vi "__uintAdd.vi"(8 "Base (decimal)":T1=10 items=["Binary"=2, "Octal"=8, "Decimal"=10, "Hexadecimal"=16, "Hexatrigesimal"=36, "ASCII"=64], 10 "Uint2 in":u8[](array[numeric])=[0], 11 "Uint1 in":u8[](array[numeric])=[0]) -> (0 "Timing":u32, 3 "Uint1 + Uint2":u8[](array[numeric]))   [LabVIEW 2011, in "UintClass.lvclass"]
uses:
  UintClass.lvclass
  enumBase.ctl
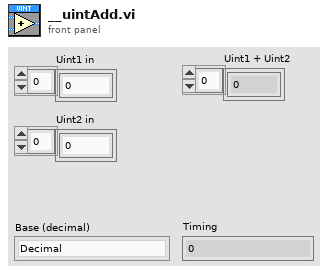
[diagram p1: front panel]
types:
  T1 = typedef "UintClass.lvclass/enumBase.ctl" = u16
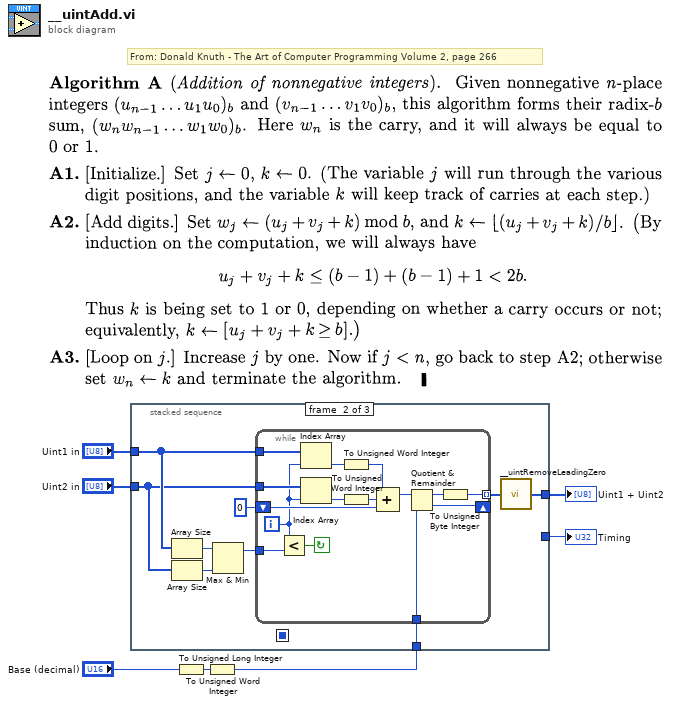
[diagram p0: block diagram]
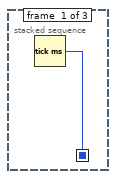
[diagram p2: hidden frame]
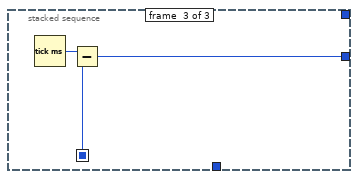
[diagram p3: hidden frame]
diagram:
  # "From: Donald Knuth - The Art of Computer Programming Volume 2, page 266"
  n1 = To Unsigned Long Integer(number="Base (decimal)") -> (unsigned 32bit integer=w4:u32)
  n2 = To Unsigned Word Integer(number=w4) -> (unsigned 16bit integer=w3:u16)
  n3 = stacked-sequence {
    seq-local: [w8 _ _] -> [_ _ w34]
    tunnel: "Uint1 in" -> [_ w15 _]
    tunnel: "Uint2 in" -> [_ w14 _]
    tunnel: [_ w12 _] -> w7
    tunnel: w3 -> [_ w10 _]
    tunnel: [_ _ w33] -> w1
    frame #0 {
      n4 = Tick Count (ms)() -> (millisecond timer value=w8:u32)
    }
    frame #1 {
      n5 = Array Size(array=w15) -> (size(s)=w17:i32)
      n6 = Array Size(array=w14) -> (size(s)=w16:i32)
      n7 = Max & Min(x=w17, y=w16) -> (max(x,y)=w9:i32)  [unwired: 1 out]
      n8 = while {
        tunnel: w15 -> [w32]
        tunnel: w14 -> [w31]
        shift-right: [w20] -> _
        shift-left: u16 0 -> [w28]
        tunnel: w9 -> [w26]
        tunnel: [w24] -> w13 mode=indexing
        tunnel: w10 -> [w19]
        i -> [w27]
        stop <- w18 continue-if-true
        n9 = Less?(x=w27, y=w26) -> (x < y?=w18:bool)
        n10 = Index Array(array=w32, index=w27) -> (element=w30:u8)
        n11 = Index Array(array=w31, index=w27) -> (element=w29:u8)
        n12 = To Unsigned Word Integer(number=w30) -> (unsigned 16bit integer=w23:u16)
        n13 = To Unsigned Word Integer(number=w29) -> (unsigned 16bit integer=w22:u16)
        n14 = Compound Arithmetic op=ADD(w23, w22, w28) -> (w21:u16)
        n15 = Quotient & Remainder(x=w21, y=w19) -> (x-y*floor(x/y)=w25:u16, floor(x/y)=w20:u16)
        n16 = To Unsigned Byte Integer(number=w25) -> (unsigned 8bit integer=w24:u8)
      }
      n17 = call "__uintRemoveLeadingZero.vi"("Uint in"=w13) -> ("Uint out"=w12:u8[])
    }
    frame #2 {
      n18 = Tick Count (ms)() -> (millisecond timer value=w35:u32)
      n19 = Subtract(x=w35, y=w34) -> (x-y=w33:u32)
    }
  }
  "Timing" <- w1
  "Uint1 + Uint2" <- w7
